vi "Laser-Main-2018-05-05.vi"() -> ()   [LabVIEW 2013]
doc: "Use this template to build a user interface event handler design pattern. Use this pattern for dialog boxes and other user interfaces. You also can create and execute user-defined events that the VI can handle the same way as user interface events."
uses:
  <vilib>/Instr/_visa.llb/VISA Configure Serial Port (Instr).vi
panel:
  in  "OFF_Laser":bool
  out "Energy":string
  out "ReturnState":string
  in  "ShutDownSystem":bool
  out "ReturnShortState":string
  out "ShortState":string
  out "LaserState":bool[](array[boolean])
  out "hex integer string":string
  out "EnergyCommand":string
  out "HVCommand":string
  out "FreqCommand":string
  in  "SetLaserEnergy":dbl=0.8
  in  "LaserHV":u8=20
  in  "LaserFreq":u8=60
  out "LaserEnergy uJ":dbl
  in  "ComForLaser":refnum<visa-resource-name>="COM3"
  in  "Serial Settings":T1={"baud rate"=9600, "data bits"=8, "parity"=enum."None", "stop bits"=10, "flow control"=0} {"flow control" items=["None"=0, "XON/XOFF"=1, "RTS/CTS"=2, "DTR/DSR"=4]; "stop bits" items=["1.0"=10, "1.5"=15, "2.0"=20]; "data bits" min=5 max=8 step=1; "baud rate" items=["75"=75, "110"=110, "134"=134, "150"=150, "300"=300, "600"=600, "1200"=1200, "1800"=1800, "2400"=2400, "4800"=4800, "7200"=7200, "9600"=9600, "14400"=14400, "19200"=19200, "28800"=28800, "38400"=38400, "56000"=56000, "57600"=57600, "115200"=115200, "128000"=128000, "230400"=230400]}
  in  "Stop_Laser":bool
  in  "Start_Laser":bool
  # "连接"
  # "待机"
  # "发射"
  # "内存"
  # "测能"
  # "温警"
  # "静态"
  # "操作"
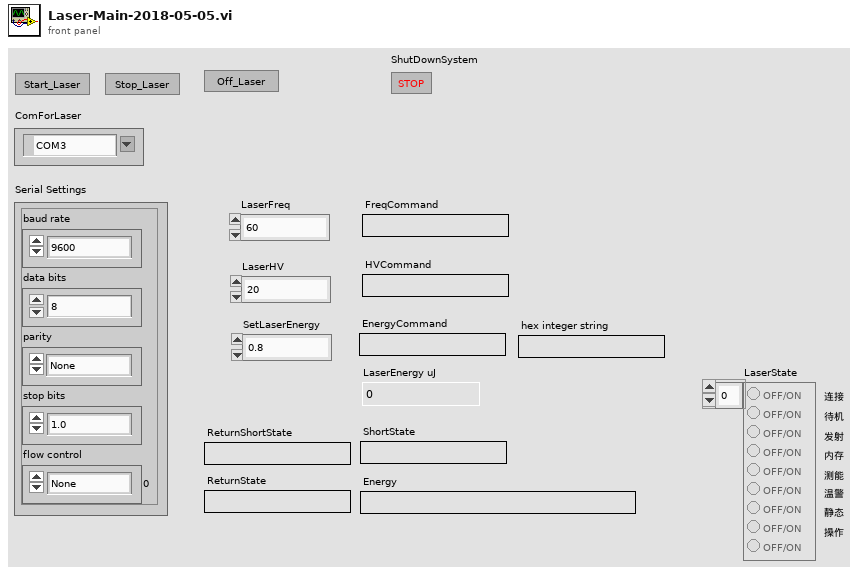
[diagram p1: front panel]
types:
  T1 = cluster{"baud rate":u32, "data bits":u16, "parity":enum16{"None", "Odd", "Even", "Mark", "Space"}, "stop bits":u16, "flow control":u16}
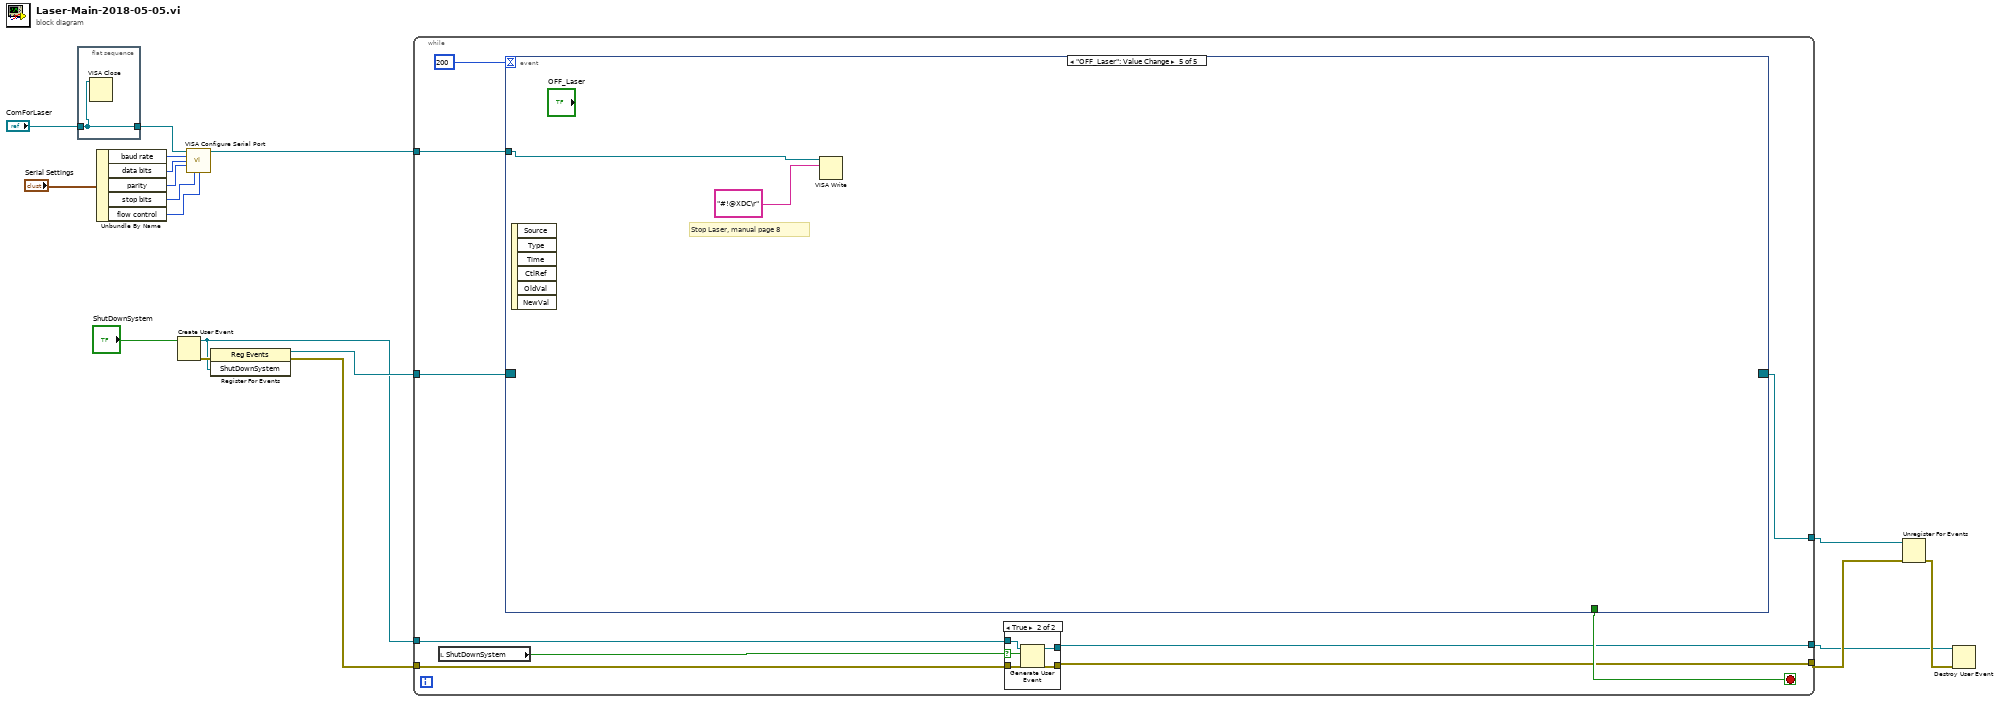
[diagram p0: block diagram]
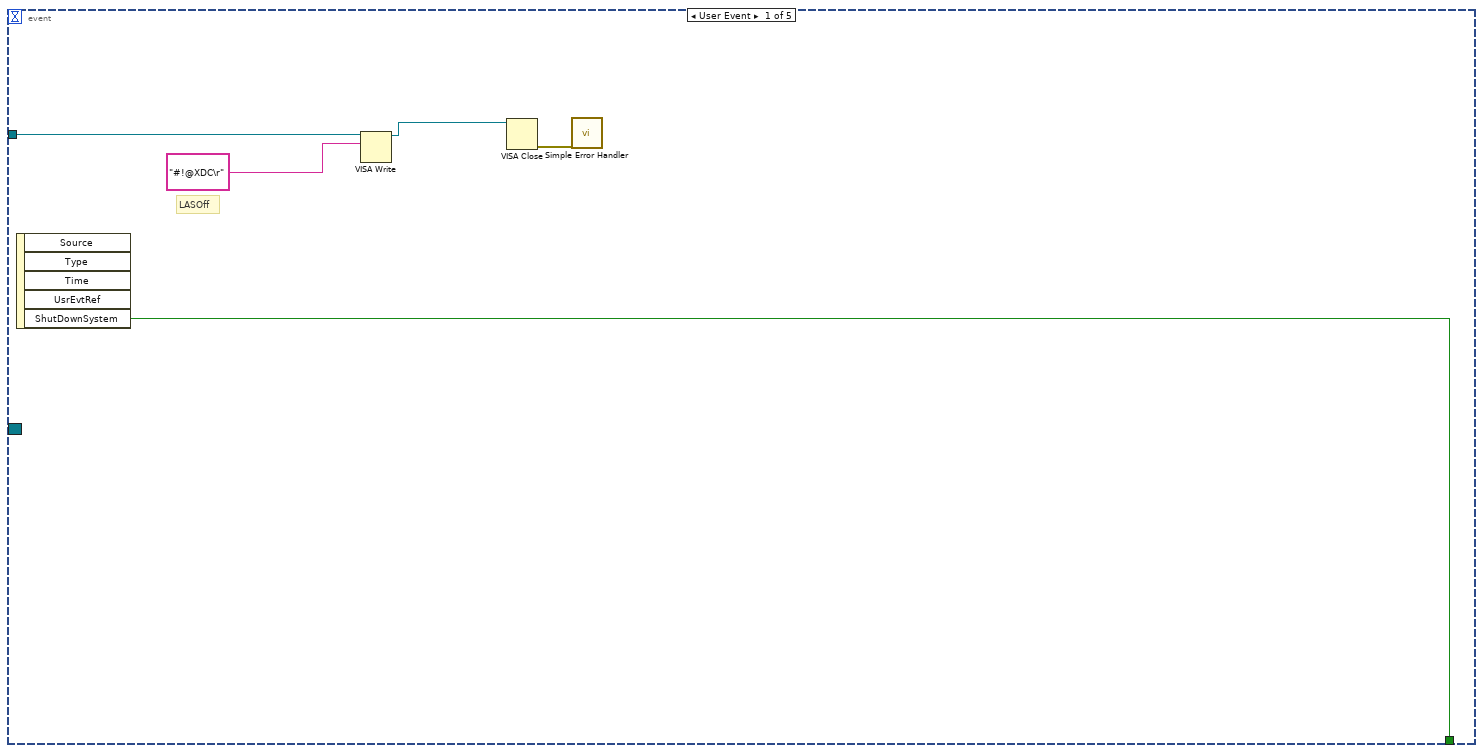
[diagram p3: hidden frame]
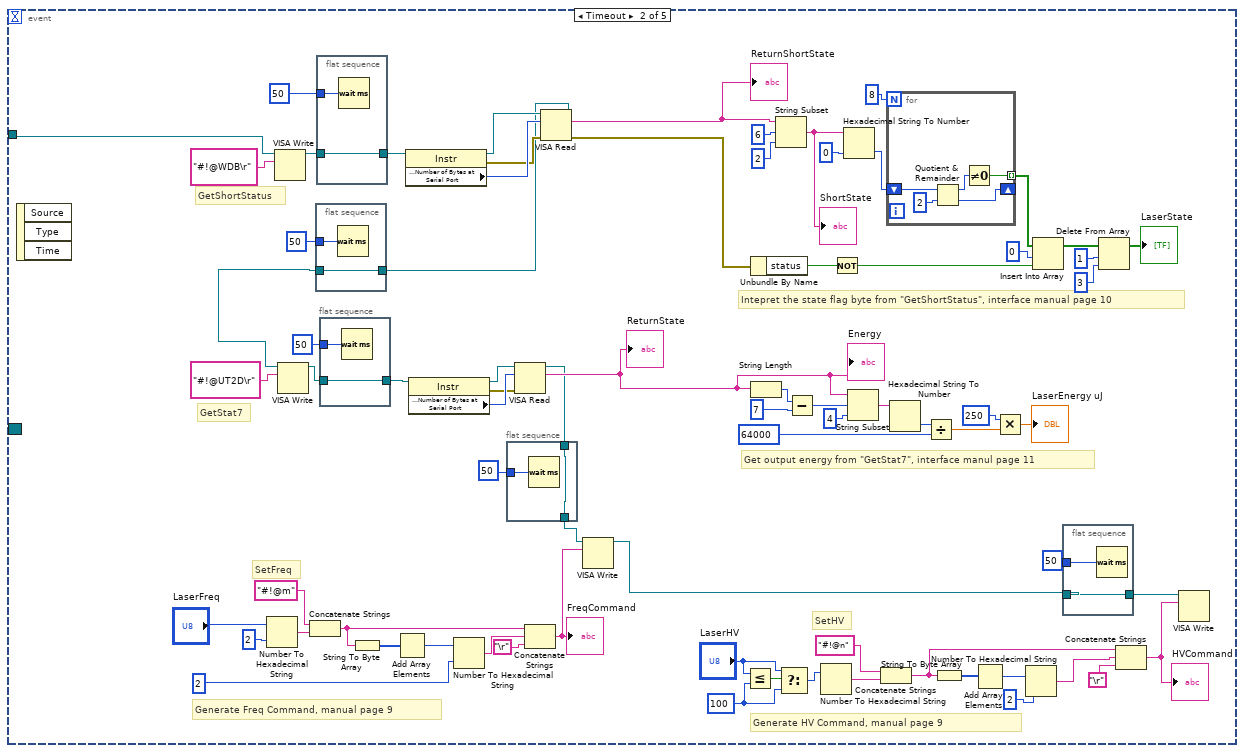
[diagram p4: hidden frame]
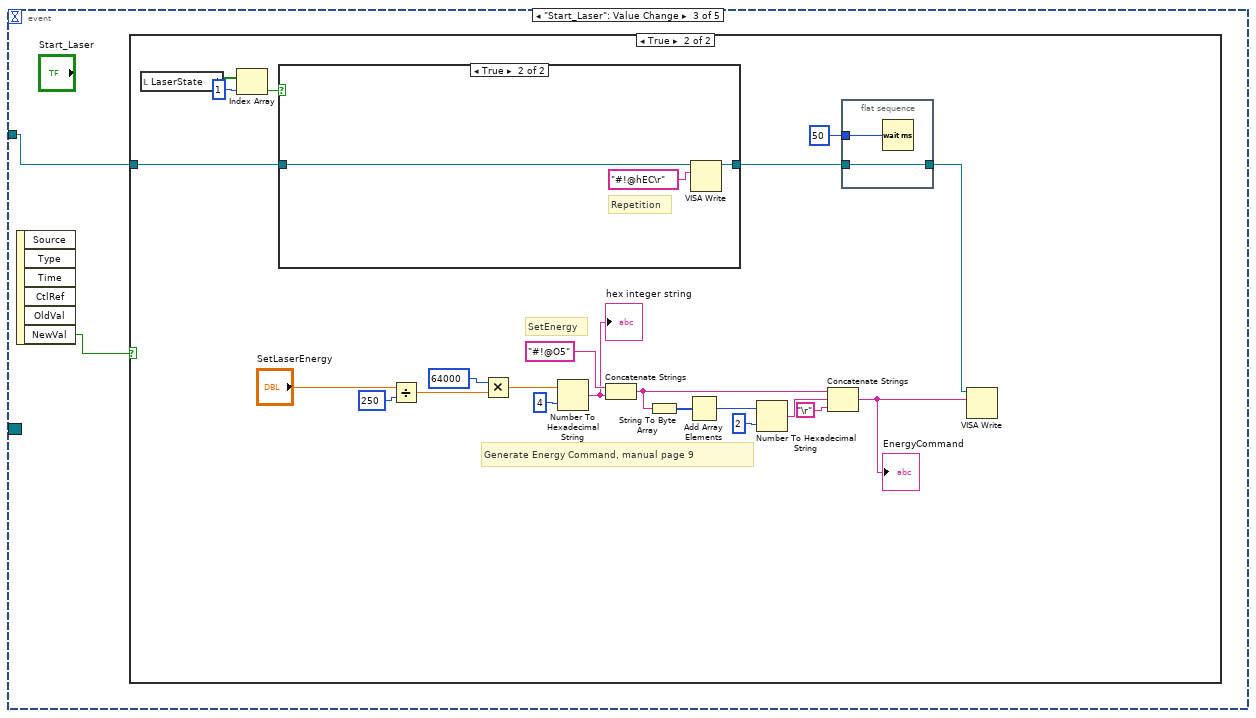
[diagram p5: hidden frame]
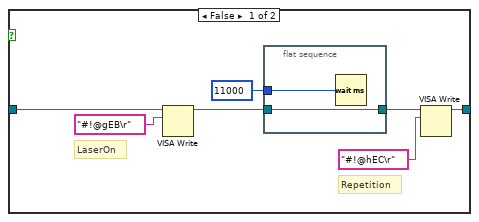
[diagram p7: hidden frame]
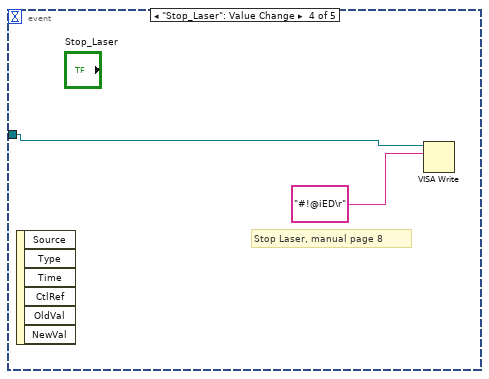
[diagram p8: hidden frame]
diagram:
  n1 = flat-sequence {
    tunnel: "ComForLaser" -> [w19]
    tunnel: [w19] -> w11
    frame #0 {
      n2 = VISA Close(VISA resource name=w19) -> ()  [unwired: 1 in, 1 out]
    }
  }
  n3 = Unbundle By Name("Serial Settings") -> ("baud rate"=w17:u32, "data bits"=w16:u16, "parity"=w15:enum16{"None", "Odd", "Even", "Mark", "Space"}, "stop bits"=w14:u16, "flow control"=w13:u16)
  n4 = Create User Event(user event datatype="ShutDownSystem") -> (user event=w5:refnum<user-event>, error out=w7:errorcluster)  [unwired: 1 in]
  n5 = call-poly "VISA Configure Serial Port"("VISA resource name"=w11, "baud rate (9600)"=w17, "data bits (8)"=w16, "parity (0:none)"=w15, "stop bits (10: 1 bit)"=w14, "flow control (0:none)"=w13) -> ("VISA resource name out"=w10:refnum<visa-resource-name>)  [unwired: 3 in, 6 out]
  n6 = register-events(error in=w7, w5) -> (reference out=w8:refnum<event-registration>, error out=w6:errorcluster)  [unwired: 1 in]
  n7 = while {
    tunnel: w10 -> [w28]
    tunnel: w8 -> [w27]
    tunnel: w6 -> [w25]
    tunnel: w5 -> [w24]
    tunnel: [w22] -> w4
    tunnel: [w21] -> w3
    tunnel: [w20] -> w1
    stop <- w23 stop-if-true
    n8 = local read "ShutDownSystem"() -> (w26:bool)
    n9 = event shown="[4] \"OFF_Laser\": Value Change" {
      selector: w27 -> [_ _ _ _ _]
      dyn-events: [_ _ _ _ _] -> w22
      timeout: 200 -> [_ _ _ _ _]
      tunnel: w28 -> [w38 w44 w133 w170 w172]
      tunnel: [w37 _ _ _ _] -> w23
      event User Event {
        # "LASOff"
        n10 = event-data() -> ("ShutDownSystem"=w37:bool)  [unwired: 1 in, 4 out]
        n11 = VISA Write(VISA resource name=w38, write buffer="#!@XDC\r") -> (VISA resource name out=w41:refnum<visa-resource-name>)  [unwired: 1 in, 2 out]
        n12 = VISA Close(VISA resource name=w41) -> (error out=w39:errorcluster)  [unwired: 1 in]
        n13 = call <vilib>:"Simple Error Handler.vi"("error in (no error)"=w39) -> ()  [unwired: 1 in, 8 out]
      }
      event Timeout {
        w71 = u8 100 ("y")
        # "Generate HV Command, manual page 9"
        # "Generate Freq Command, manual page 9"
        # "Get output energy from \"GetStat7\", interface manul page 11"
        # "Intepret the state flag byte from \"GetShortStatus\", interface manual page 10"
        # "SetHV"
        # "SetFreq"
        # "GetStat7"
        # "GetShortStatus"
        n14 = event-data() -> ()  [unwired: 1 in, 3 out]
        n15 = Number To Hexadecimal String(1:i16 2 ("width (-)"), 2:"LaserFreq") -> (0:w85:string)
        n16 = VISA Write(VISA resource name=w44, write buffer="#!@WDB\r") -> (VISA resource name out=w111:refnum<visa-resource-name>)  [unwired: 1 in, 2 out]
        n17 = VISA Write(VISA resource name=w76, write buffer="#!@UT2D\r") -> (VISA resource name out=w101:refnum<visa-resource-name>)  [unwired: 1 in, 2 out]
        n18 = Concatenate Strings("#!@m" ("string"), w85) -> (w81:string)
        n19 = flat-sequence {
          tunnel: [w124] -> w76
          tunnel: w77 -> [w124]
          tunnel: u32 50 ("delay before read (ms)") -> [w125]
          frame #0 {
            n20 = Wait (ms)(milliseconds to wait=w125) -> ()  [unwired: 1 out]
          }
        }
        n21 = flat-sequence {
          tunnel: w111 -> [w130]
          tunnel: [w130] -> w112
          tunnel: u32 50 ("delay before read (ms)") -> [w131]
          frame #0 {
            n22 = Wait (ms)(milliseconds to wait=w131) -> ()  [unwired: 1 out]
          }
        }
        n23 = flat-sequence {
          tunnel: w101 -> [w128]
          tunnel: [w128] -> w102
          tunnel: u32 50 ("delay before read (ms)") -> [w129]
          frame #0 {
            n24 = Wait (ms)(milliseconds to wait=w129) -> ()  [unwired: 1 out]
          }
        }
        n25 = String To Byte Array(string=w81) -> (unsigned byte array=w84:u8[])
        n26 = Add Array Elements(numeric array=w84) -> (sum=w83:u8)
        n27 = property class="Instr"(reference=w112) -> (reference out=w113:refnum<visa-resource-name>, error out=w114:errorcluster, "Serial Settings:Number of Bytes at Serial Port"=w115:u32)  [unwired: 1 in]
        n28 = property class="Instr"(reference=w102) -> (reference out=w103:refnum<visa-resource-name>, error out=w104:errorcluster, "Serial Settings:Number of Bytes at Serial Port"=w105:u32)  [unwired: 1 in]
        n29 = Number To Hexadecimal String(1:i16 2 ("width (-)"), 2:w83) -> (0:w80:string)
        n30 = flat-sequence {
          tunnel: u32 50 ("delay before read (ms)") -> [w127]
          tunnel: w43 -> [w126]
          tunnel: [w126] -> w42
          frame #0 {
            n31 = Wait (ms)(milliseconds to wait=w127) -> ()  [unwired: 1 out]
          }
        }
        n32 = VISA Read(VISA resource name=w103, byte count=w105, error in (no error)=w104) -> (VISA resource name out=w43:refnum<visa-resource-name>, read buffer=w96:string)  [unwired: 2 out]
        "ReturnState" <- w96
        "Energy" <- w96
        n33 = Concatenate Strings(w81, w80, "\r") -> (w74:string)
        "FreqCommand" <- w74
        n34 = VISA Read(VISA resource name=w113, byte count=w115, error in (no error)=w114) -> (VISA resource name out=w77:refnum<visa-resource-name>, read buffer=w109:string, error out=w56:errorcluster)  [unwired: 1 out]
        "ReturnShortState" <- w109
        n35 = VISA Write(VISA resource name=w42, write buffer=w74) -> (VISA resource name out=w60:refnum<visa-resource-name>)  [unwired: 1 in, 2 out]
        n36 = Less Or Equal?(x="LaserHV", y=w71) -> (x <= y?=w73:bool)
        n37 = Unbundle By Name(w56) -> ("status"=w55:bool)
        n38 = String Length(string=w96) -> (length=w99:i32)
        n39 = String Subset(string=w109, offset (0)=6, length (rest)=2 ("length (rest)")) -> (substring=w48:string)
        "ShortState" <- w48
        n40 = Select(t="LaserHV", s=w73, f=w71) -> (s? t:f=w62:u8)
        n41 = Subtract(x=w99, y=7) -> (x-y=w97:i32)
        n42 = Number To Hexadecimal String(2:w62) -> (0:w69:string)  [unwired: 1 in]
        n43 = Not(x=w55) -> (.not. x?=w54:bool)
        n44 = Hexadecimal String To Number(string=w48, default (0uL)=u8 0 ("default (0 U32)")) -> (number=w49:u8)  [unwired: 1 in, 1 out]
        n45 = String Subset(string=w96, offset (0)=w97, length (rest)=4) -> (substring=w94:string)
        n46 = Concatenate Strings("#!@n" ("string"), w69) -> (w65:string)
        n47 = for {
          N: 8 -> [_]
          tunnel: [w119] -> w45 mode=indexing
          shift-right: [w118] -> _
          shift-left: w49 -> [w117]
          n48 = Quotient & Remainder(x=w117, y=2) -> (x-y*floor(x/y)=w120:i32, floor(x/y)=w118:i32)
          n49 = Not Equal To 0?(x=w120) -> (x != 0?=w119:bool)
        }
        n50 = Hexadecimal String To Number(string=w94) -> (number=w93:u32)  [unwired: 2 in, 1 out]
        n51 = Divide(x=w93, y=u32 64000) -> (x/y=w91:dbl)
        n52 = String To Byte Array(string=w65) -> (unsigned byte array=w68:u8[])
        n53 = Add Array Elements(numeric array=w68) -> (sum=w67:u8)
        n54 = Multiply(x=250, y=w91) -> (x*y=→"LaserEnergy uJ":dbl)
        n55 = Number To Hexadecimal String(1:i16 2 ("width (-)"), 2:w67) -> (0:w64:string)
        n56 = Insert Into Array(array=w45, index=0, new element=w54) -> (w46:bool[])
        n57 = flat-sequence {
          tunnel: w60 -> [w122]
          tunnel: [w122] -> w59
          tunnel: u32 50 ("delay before read (ms)") -> [w123]
          frame #0 {
            n58 = Wait (ms)(milliseconds to wait=w123) -> ()  [unwired: 1 out]
          }
        }
        n59 = Delete From Array(array=w46, length=1, index=3) -> (array with subset deleted=→"LaserState":bool[])  [unwired: 1 out]
        n60 = Concatenate Strings(w65, w64, "\r") -> (w58:string)
        "HVCommand" <- w58
        n61 = VISA Write(VISA resource name=w59, write buffer=w58) -> ()  [unwired: 1 in, 3 out]
      }
      event "Start_Laser": Value Change {
        n62 = event-data() -> ("NewVal"=w132:bool)  [unwired: 1 in, 5 out]
        n63 = case shown="True" w132 {
          tunnel: w133 -> [_ w134]
          frame False {
          }
          frame True {
            # "Generate Energy Command, manual page 9"
            # "SetEnergy"
            n64 = local read "LaserState"() -> (w155:bool[])
            n65 = Index Array(array=w155, index=1) -> (element=w153:bool)
            n66 = case shown="True" w153 {
              tunnel: w134 -> [w159 w168]
              tunnel: [w158 w167] -> w136
              frame False {
                # "LaserOn"
                # "Repetition"
                n67 = VISA Write(VISA resource name=w159, write buffer="#!@gEB\r") -> (VISA resource name out=w162:refnum<visa-resource-name>)  [unwired: 1 in, 2 out]
                n68 = flat-sequence {
                  tunnel: w162 -> [w166]
                  tunnel: [w166] -> w160
                  tunnel: u32 11000 ("delay before read (ms)") -> [w165]
                  frame #0 {
                    n69 = Wait (ms)(milliseconds to wait=w165) -> ()  [unwired: 1 out]
                  }
                }
                n70 = VISA Write(VISA resource name=w160, write buffer="#!@hEC\r") -> (VISA resource name out=w158:refnum<visa-resource-name>)  [unwired: 1 in, 2 out]
              }
              frame True {
                # "Repetition"
                n71 = VISA Write(VISA resource name=w168, write buffer="#!@hEC\r") -> (VISA resource name out=w167:refnum<visa-resource-name>)  [unwired: 1 in, 2 out]
              }
            }
            n72 = Divide(x="SetLaserEnergy", y=250) -> (x/y=w141:dbl)
            n73 = Multiply(x=64000, y=w141) -> (x*y=w139:dbl)
            n74 = Number To Hexadecimal String(1:i16 4 ("width (-)"), 2:w139) -> (0:w150:string)
            "hex integer string" <- w150
            n75 = Concatenate Strings("#!@O5" ("string"), w150) -> (w146:string)
            n76 = String To Byte Array(string=w146) -> (unsigned byte array=w149:u8[])
            n77 = Add Array Elements(numeric array=w149) -> (sum=w148:u8)
            n78 = Number To Hexadecimal String(1:i16 2 ("width (-)"), 2:w148) -> (0:w145:string)
            n79 = Concatenate Strings(w146, w145, "\r") -> (w137:string)
            "EnergyCommand" <- w137
            n80 = flat-sequence {
              tunnel: u32 50 ("delay before read (ms)") -> [w157]
              tunnel: w136 -> [w156]
              tunnel: [w156] -> w135
              frame #0 {
                n81 = Wait (ms)(milliseconds to wait=w157) -> ()  [unwired: 1 out]
              }
            }
            n82 = VISA Write(VISA resource name=w135, write buffer=w137) -> ()  [unwired: 1 in, 3 out]
          }
        }
      }
      event "Stop_Laser": Value Change {
        # "Stop Laser, manual page 8"
        n83 = event-data() -> ()  [unwired: 1 in, 6 out]
        n84 = VISA Write(VISA resource name=w170, write buffer="#!@iED\r") -> ()  [unwired: 1 in, 3 out]
      }
      event "OFF_Laser": Value Change {
        # "Stop Laser, manual page 8"
        n85 = event-data() -> ()  [unwired: 1 in, 6 out]
        n86 = VISA Write(VISA resource name=w172, write buffer="#!@XDC\r") -> ()  [unwired: 1 in, 3 out]
      }
    }
    n87 = case shown="True" w26 {
      selector: w26 -> [_ w34]
      tunnel: w25 -> [w30 w36]
      tunnel: w24 -> [w31 w35]
      tunnel: [w30 w33] -> w21
      tunnel: [w31 w32] -> w20
      frame False {
      }
      frame True {
        n88 = Generate User Event(user event=w35, event data cluster=w34, error in=w36) -> (user event out=w32:refnum<user-event>, error out=w33:errorcluster)  [unwired: 1 in]
      }
    }
  }
  n89 = Unregister For Events(event registration refnum=w4, error in=w3) -> (error out=w2:errorcluster)
  n90 = Destroy User Event(user event=w1, error in=w2) -> ()  [unwired: 1 out]
